vi "OpenByteStreamFileForWriting.vi"(0 "Path":path) -> (1 "Byte Stream File Refnum":refnum<file>, 2 "error out":errorcluster)   [LabVIEW 2011]
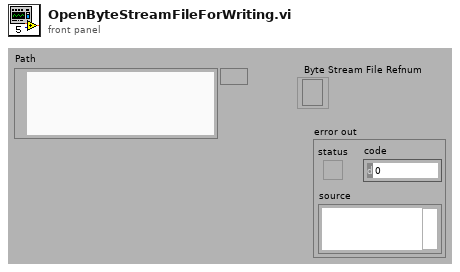
[diagram p1: front panel]
types:
  T1 = enum16{"open", "replace", "create", "open or create", "replace or create", "replace or create with confirmation"}
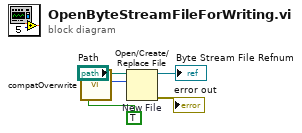
[diagram p0: block diagram]
diagram:
  n1 = call <vilib>:"compatOverwrite.vi"("overwrite (F)"=TRUE) -> ("overwrite?"=w1:T1)
  n2 = Open/Create/Replace File "New File"(file path (use dialog)="Path", operation (0:open)=w1) -> (refnum out=→"Byte Stream File Refnum":refnum<file>, error out=→"error out":errorcluster)  [unwired: 1 in, 4 out]
